vi "HealthCheckUI.vi"(8 "Enum in":T1, 9 "Edit Table":bool, 10 "Table in":refnum<vi>, 11 "HealthCheck.lvclass":refnum<class "HealthCheck.lvclass">) -> (0 "Enum out":T1, 3 "HealthCheck out":refnum<class "HealthCheck.lvclass">)   [LabVIEW 2018, in "HealthCheck.lvclass"]
uses:
  HealthCheck.lvclass
  HCState_TypeDef.ctl
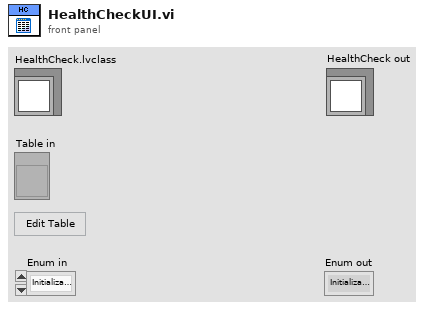
[diagram p1: front panel]
types:
  T1 = typedef "HealthCheck.lvclass/HCState_TypeDef.ctl" = enum16{"Initialization", "Running", "Modify Table"}
  T2 = enum32{"Invalid", "Standard", "Closed", "Hidden", "Minimized", "Maximized"}
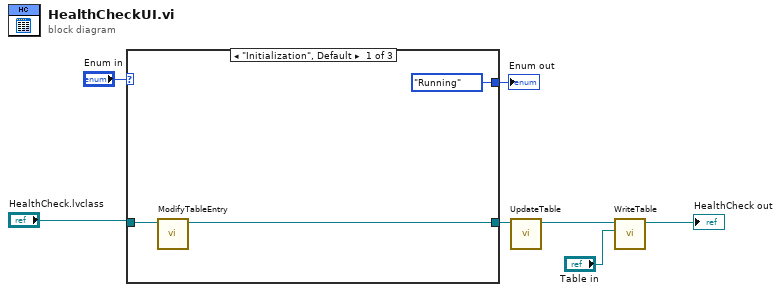
[diagram p0: block diagram]
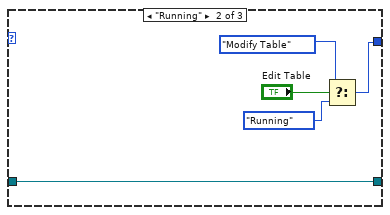
[diagram p2: hidden frame]
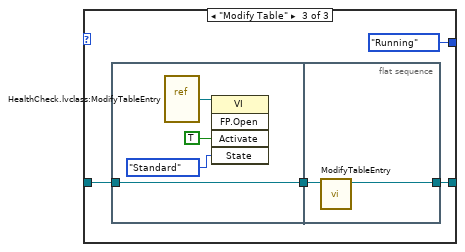
[diagram p3: hidden frame]
diagram:
  n1 = case shown="\"Initialization\", Default" "Enum in" {
    tunnel: [HCState_TypeDef."Running" w15 HCState_TypeDef."Running"] -> w2
    tunnel: [w9 w11 w18] -> w6
    tunnel: "HealthCheck.lvclass" -> [w8 w11 w16]
    frame "Initialization", Default {
      n2 = call "ModifyTableEntry.vi"("HealthCheck in"=w8) -> ("HealthCheck out"=w9:refnum<class "HealthCheck.lvclass">)  [unwired: 9 in, 1 out]
    }
    frame "Running" {
      n3 = Select(t=HCState_TypeDef."Modify Table", s="Edit Table", f=HCState_TypeDef."Running") -> (s? t:f=w15:T1)
    }
    frame "Modify Table" {
      n4 = flat-sequence {
        tunnel: [w20] -> w17
        tunnel: w16 -> [w20]
        tunnel: [w25] -> w18
        tunnel: w17 -> [w24]
        frame #0 {
          n5 = vi-ref "HealthCheck.lvclass:ModifyTableEntry.vi"() -> (w23:refnum<vi>)
          n6 = invoke class="VI" method="FP.Open"(reference=w23, "Activate"=TRUE ("Activate?"), "State"=T2."Standard") -> ()  [unwired: 2 in, 5 out]
        }
        frame #1 {
          n7 = call "ModifyTableEntry.vi"("HealthCheck in"=w24) -> ("HealthCheck out"=w25:refnum<class "HealthCheck.lvclass">)  [unwired: 9 in, 1 out]
        }
      }
    }
  }
  "Enum out" <- w2
  n8 = call "UpdateTable.vi"("HealthCheck in"=w6) -> ("HealthCheck out"=w5:refnum<class "HealthCheck.lvclass">)  [unwired: 9 in, 1 out]
  n9 = call "WriteTable.vi"("Table in"="Table in", "HealthCheck in"=w5) -> ("HealthCheck out"=→"HealthCheck out":refnum<class "HealthCheck.lvclass">)  [unwired: 8 in, 1 out]
